vi "Solve1.vi"(8 "Error In":errorcluster, 11 "object in":refnum<class "2024_13.lvclass">) -> (0 "Error Out":errorcluster, 2 "Result":u64, 3 "object out":refnum<class "2024_13.lvclass">)   [LabVIEW 2023, in "2024_13.lvclass"]
uses:
  2024_13.lvclass
  Game.ctl
  Common/AOC_XY.ctl
  2024_13.lvclass/2024_13.ctl
  <vilib>/Analysis/7linalg.llb/Solve Linear Equations (single right hand).vi
  <vilib>/Analysis/baseanly.llb/Solve Linear Equations By Cholesky.vi
  <vilib>/Analysis/baseanly.llb/Real Matrix to Compact Array.vi
  <vilib>/Analysis/baseanly.llb/Real Compact Tri-Matrix Linear Eqs.vi
  <vilib>/Analysis/7linalg.llb/Solve Linear Eqs (General).vi
  <vilib>/Analysis/7linalg.llb/Solve Linear Eqs (Gen, single right hand).vi
  <vilib>/Analysis/NI_AALPro.lvlib
panel:
  out "Array":dbl[](array[numeric])
  out "Solution Vector":dbl[](array[numeric]) format="%.2f"
  out "Games":T1[](array[typedef])
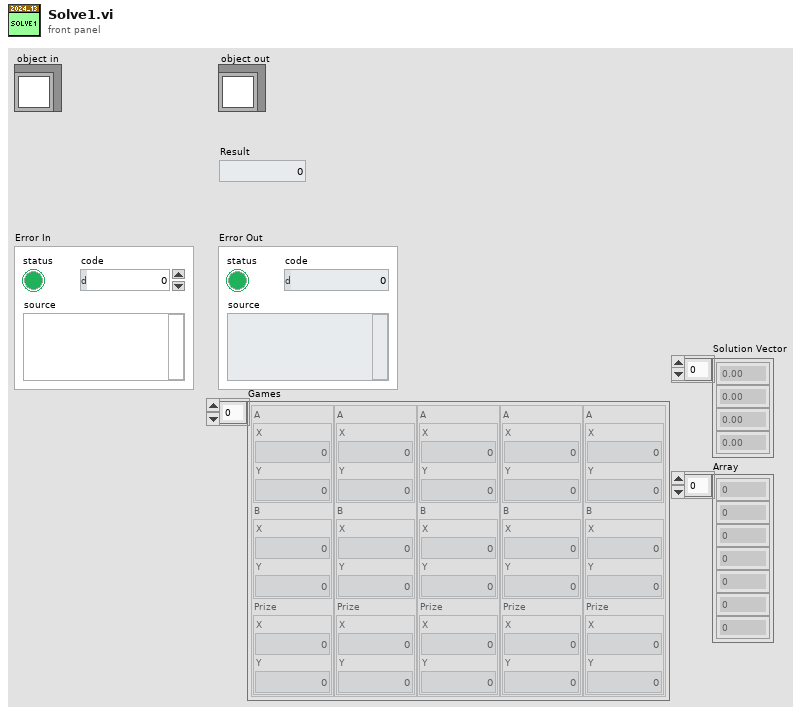
[diagram p1: front panel]
types:
  T1 = typedef "2024_13.lvclass/Game.ctl" = cluster{"A":T2, "B":T2, "Prize":T2}
  T2 = typedef "AOC_XY.ctl" = cluster{"X":u64, "Y":u64}
  T3 = typedef "NI_Matrix.lvlib/RealMatrix.ctl" = dbl[][]
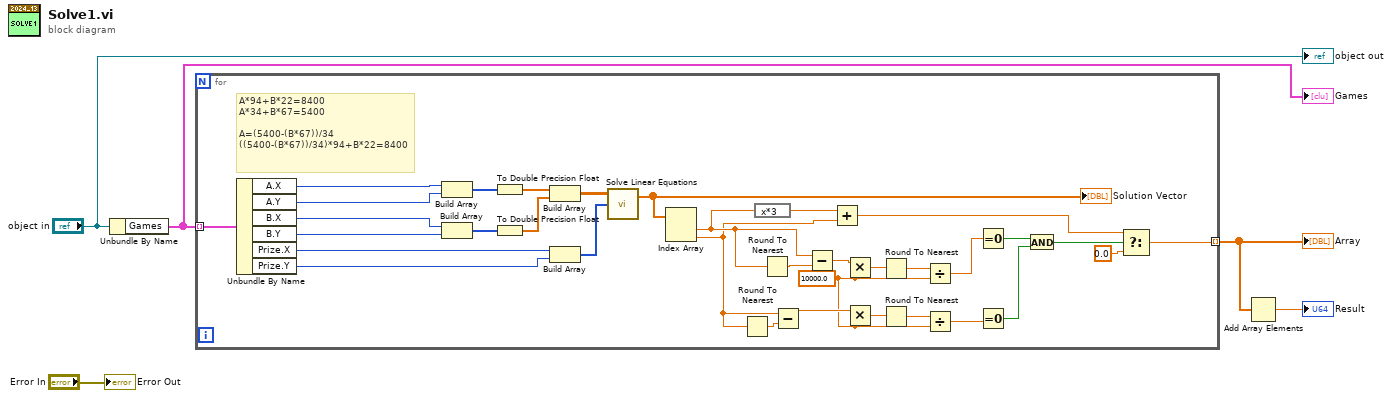
[diagram p0: block diagram]
diagram:
  n1 = Unbundle By Name("object in") -> ("Games"=w3:T1[])
  "Games" <- w3
  n2 = for {
    tunnel: w3 -> [w39] mode=indexing
    tunnel: [w19] -> w2 mode=indexing
    w7 = 10000.0 ("y")
    # "A*94+B*22=8400\nA*34+B*67=5400\n\nA=(5400-(B*67))/34\n((5400-(B*67))/34)*94+B*22=8400"
    n3 = Unbundle By Name(w39) -> ("A.X"=w38:u64, "A.Y"=w28:u64, "B.X"=w27:u64, "B.Y"=w37:u64, "Prize.X"=w31:u64, "Prize.Y"=w30:u64)
    n4 = Build Array(w38, w28) -> (w36:u64[])
    n5 = Build Array(w27, w37) -> (w35:u64[])
    n6 = To Double Precision Float(number=w36) -> (double precision float=w34:dbl[])
    n7 = To Double Precision Float(number=w35) -> (double precision float=w33:dbl[])
    n8 = Build Array(w34, w33) -> (w32:T3)
    n9 = Build Array(w31, w30) -> (w29:u64[])
    n10 = call-poly <vilib>:"Solve Linear Equations.vi"("Known Vector"=w29, "Input Matrix"=w32) -> ("Solution Vector"=w26:dbl[])  [unwired: 1 in, 1 out]
    "Solution Vector" <- w26
    n11 = Index Array(array=w26) -> (element #1=w16:dbl, element #2=w15:dbl)  [unwired: 2 in]
    n12 = Round To Nearest(number=w15) -> (nearest integer value=w17:dbl)
    n13 = expression code="x*3"(w16) -> (w25:dbl)
    n14 = Round To Nearest(number=w16) -> (nearest integer value=w18:dbl)
    n15 = Subtract(x=w15, y=w17) -> (x-y=w8:dbl)
    n16 = Subtract(x=w16, y=w18) -> (x-y=w14:dbl)
    n17 = Add(x=w25, y=w15) -> (x+y=w21:dbl)
    n18 = Multiply(x=w14, y=w7) -> (x*y=w13:dbl)
    n19 = Multiply(x=w8, y=w7) -> (x*y=w9:dbl)
    n20 = Round To Nearest(number=w13) -> (nearest integer value=w12:dbl)
    n21 = Round To Nearest(number=w9) -> (nearest integer value=w10:dbl)
    n22 = Divide(x=w12, y=w7) -> (x/y=w11:dbl)
    n23 = Divide(x=w10, y=w7) -> (x/y=w6:dbl)
    n24 = Equal To 0?(x=w11) -> (x = 0?=w24:bool)
    n25 = Equal To 0?(x=w6) -> (x = 0?=w23:bool)
    n26 = And(x=w24, y=w23) -> (x .and. y?=w22:bool)
    n27 = Select(t=w21, s=w22, f=0.0 ("y")) -> (s? t:f=w19:dbl)
  }
  "Array" <- w2
  n28 = Add Array Elements(numeric array=w2) -> (sum=→"Result":dbl)
  "Error Out" <- "Error In"
  "object out" <- "object in"
